vi "DisplayTemperaturesFVIR.vi"(0 "Array":string[](array[string])) -> (7 "FVIR array 2":string[][](array[string]), 10 "Logical OR array":bool)   [LabVIEW 2020, in "Modbus.lvlib"]
uses:
  Modbus/Modbus.lvlib
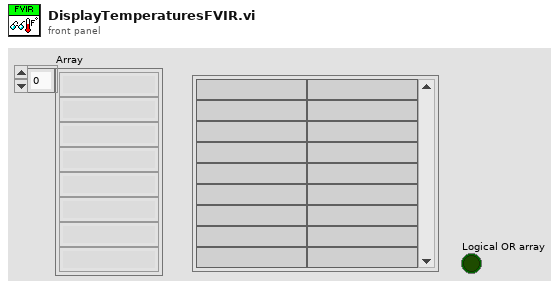
[diagram p1: front panel]
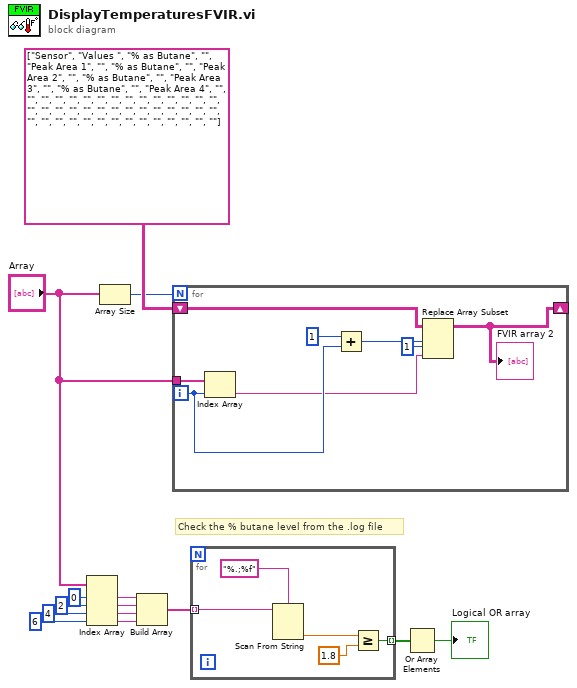
[diagram p0: block diagram]
diagram:
  # "Check the % butane level from the .log file"
  n1 = Index Array(array="Array", index #1=0 ("index"), index #2=2 ("index"), index #3=4 ("index"), index #4=6 ("index")) -> (element #1=w6:string, element #2=w5:string, element #3=w4:string, element #4=w3:string)
  n2 = Array Size(array="Array") -> (size(s)=w13:i32)
  n3 = Build Array(w6, w5, w4, w3) -> (w7:string[])
  n4 = for {
    N: w13 -> [_]
    tunnel: "Array" -> [w22]
    shift-right: [w20] -> _
    shift-left: string[][] [["Sensor", "Values "], ["% as Butane", ""], ["Peak Area 1", ""], ["% as Butane", ""], ["Peak Area 2", ""], ["% as Butane", ""], ["Peak Area 3", ""], ["% as Butane", ""], ["Peak Area 4", ""], ["", ""], ["", ""], ["", ""], ["", ""], ["", ""], ["", ""], ["", ""], ["", ""], ["", ""], ["", ""], ["", ""], ["", ""], ["", ""], ["", ""], ["", ""], ["", ""], ["", ""], ["", ""], ["", ""], ["", ""], ["", ""]] ("Array 2") -> [w21]
    i -> [w17]
    n5 = Index Array(array=w22, index=w17) -> (element=w15:string)
    n6 = Add(x=1 ("disabled index (col)"), y=w17) -> (x+y=w19:i32)
    n7 = Replace Array Subset(array=w21, new element=w15, index (row)=w19, index (col)=1 ("disabled index (col)")) -> (w20:string[][])
    "FVIR array 2" <- w20
  }
  n8 = for {
    tunnel: w7 -> [w26] mode=indexing
    tunnel: [w23] -> w2 mode=indexing
    n9 = Scan From String(format string="%.;%f", input string=w26) -> (output 1=w25:dbl)  [unwired: 3 in, 3 out]
    n10 = Greater Or Equal?(x=w25, y=1.8) -> (x >= y?=w23:bool)
  }
  n11 = Or Array Elements(Boolean array=w2) -> (logical OR=→"Logical OR array":bool)
